vi "Reset.vi"(8 "error in (no error)":errorcluster, 10 "Message in":refnum<class "ResetMessage.lvclass">, 11 "MeritFactor in":refnum<class "MeritFactor.lvclass">) -> (0 "error out":errorcluster, 3 "MeritFactor out":refnum<class "MeritFactor.lvclass">)   [LabVIEW 2012, in "MeritFactor.lvclass"]
doc: "The reset method processes the command 'reset'. \n\nResets the internal state of the component (without performing a full initialisation). This could be resetting hardware, or private data to default values."
uses:
  MeritFactor.lvclass
  <vilib>/Distrio/Murmex/ResetMessage/ResetMessage.lvclass
  <vilib>/Distrio/Murmex/Murmex/Murmex.lvclass
  MeritFactor.lvclass/MeritFactor.ctl
panel:
  # "This method is called when the RESET\ntrigger is sent. \n\nOverride this method when your component needs to\nrespond to this trigger. \n\nCall parent for proper implementation"
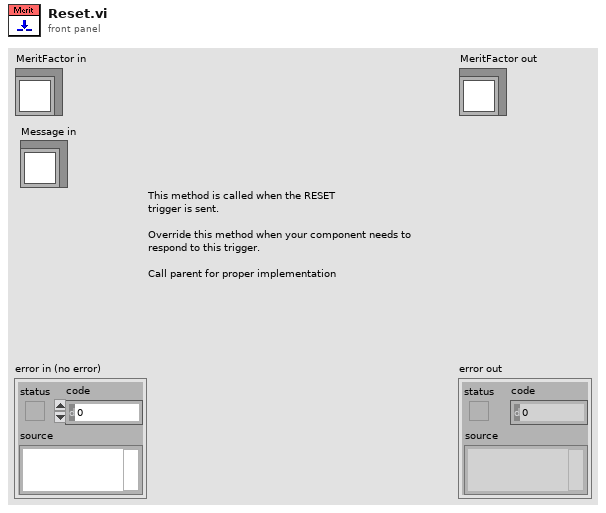
[diagram p1: front panel]
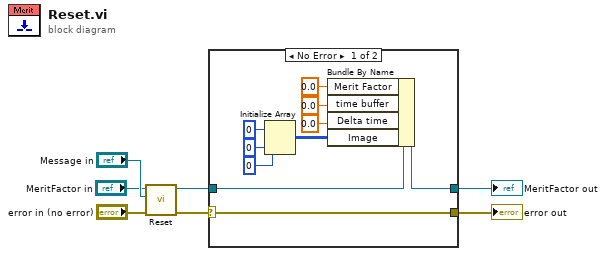
[diagram p0: block diagram]
diagram:
  n1 = call-parent "Reset.vi"("error in (no error)"="error in (no error)", "Message in"="Message in", "Murmex in"="MeritFactor in") -> ("error out"=w4:errorcluster, "Murmex out"=w3:refnum<class "MeritFactor.lvclass">)  [unwired: 7 in]
  n2 = case shown="No Error" w4 {
    selector: w4 -> [w15 w18]
    tunnel: w3 -> [w17 w19]
    tunnel: [w16 w19] -> w2
    tunnel: [w15 w18] -> w1
    frame No Error {
      n3 = Initialize Array(u16 0 ("element"), 0 ("dimension size"), 0 ("dimension size")) -> (w8:u16[][])
      n4 = Bundle By Name(cluster=w17, "Merit Factor"=0.0 ("settings cluster.Merit Factor"), "time buffer"=0.0 ("run-time cluster.time buffer"), "Delta time"=0.0 ("run-time cluster.Delta time"), "Image"=w8) -> (w16:refnum<class "MeritFactor.lvclass">)
    }
    frame Error {
    }
  }
  "error out" <- w1
  "MeritFactor out" <- w2
